vi "Connect.vi"(8 "error in (no error)":errorcluster caption="entrée d'erreur (pas d'erreur)", 11 "Server TCP_IP (Default) en entrée":refnum<class "Client TCP_IP (Default).lvclass">) -> (0 "error out":errorcluster caption="sortie d'erreur", 3 "Server TCP_IP (Default) en sortie":refnum<class "Client TCP_IP (Default).lvclass">)   [LabVIEW 2020, in "Library Instrument & Equipement.lvlib" / "Library TCP IP.lvlib" / "Client TCP_IP (Default).lvclass"]
uses:
  Client TCP_IP (Default).lvclass
  Client TCP_IP (Default).lvclass/Client TCP_IP (Default).ctl
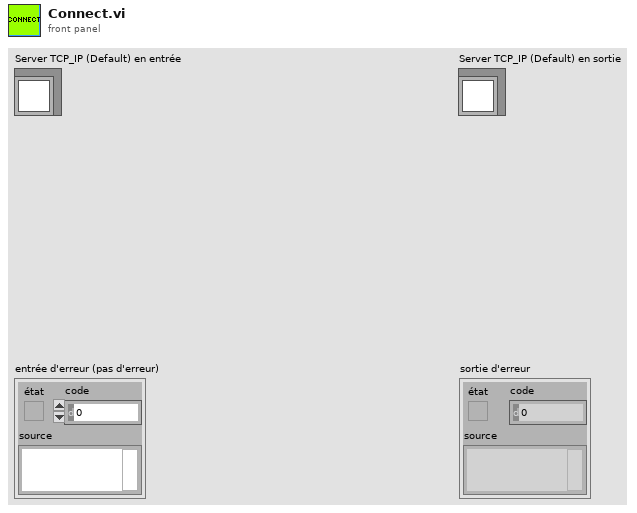
[diagram p1: front panel]
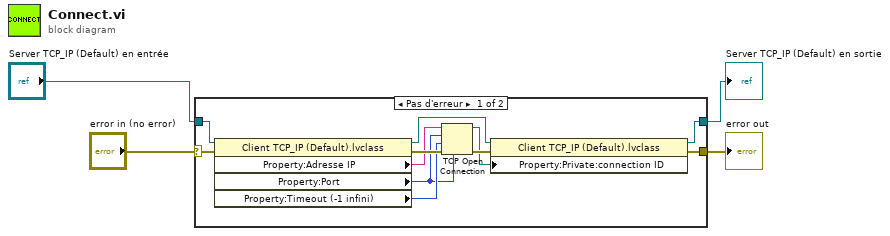
[diagram p0: block diagram]
diagram:
  n1 = case shown="Pas d'erreur" "error in (no error)" {
    selector: "error in (no error)" -> [w7 w17]
    tunnel: [w13 w17] -> w3
    tunnel: [w8 w16] -> w1
    tunnel: "Server TCP_IP (Default) en entrée" -> [w15 w16]
    frame No Error {
      n2 = property class="Client TCP_IP (Default).lvclass"(reference=w15, error in=w7) -> (reference out=w14:refnum<class "Client TCP_IP (Default).lvclass">, error out=w11:errorcluster, "Property:Adresse IP"=w6:string, "Property:Port"=w5:u16, "Property:Timeout (-1 infini)"=w9:i16)
      n3 = TCP Open Connection(address=w6, remote port or service name=w5, timeout ms (60000)=w9, local port=w5, error in (no error)=w11) -> (connection ID=w10:refnum<k5>, error out=w12:errorcluster)
      n4 = property class="Client TCP_IP (Default).lvclass"(reference=w14, error in=w12, "Property:Private:connection ID"=w10) -> (reference out=w8:refnum<class "Client TCP_IP (Default).lvclass">, error out=w13:errorcluster)
    }
    frame Error {
    }
  }
  "error out" <- w3
  "Server TCP_IP (Default) en sortie" <- w1
